vi "Tool_Playground.vi"() -> ()   [LabVIEW 2019]
uses:
  Parse/ParseVectorFile/Typedefs/PublicEvents--ParseVectorFile.ParsedData.ctl
  Parse/Image/SVGImage.lvclass
  Parse/ParsePaths/Path.lvclass
  Parse/Rectangle/Rectangle.lvclass
  Parse/Dot/Dot.lvclass
  Parse/ParseVectorFile/ParseVectorFile.lvclass
  C:/Program Files (x86)/National Instruments/LabVIEW 2019/vi.lib/JKI/JKI SMO/SMO/SMO.lvclass
  Settings/Rectangle Settings/Rectangle Settings.lvclass
  C:/Users/Albro/Documents/GitHub/AFM-Lithography/lvsrc/Classes/Settings/ObjectSettings/ObjectSettings.lvclass
  subVIs/typedefs/Schedule Types/Schedule--Constant.ctl
  Settings/ObjectSettings/ObjectSettings.lvclass/ObjectSettings.ctl
  Settings/Rectangle Settings/Rectangle Settings.lvclass/Rectangle Settings.ctl
  Settings/ObjectSettings/Accessors/Write Direction.vi
  Settings/ObjectSettings/Accessors/Write Enabled.vi
  Settings/ObjectSettings/Accessors/Write Resistance.vi
  Settings/ObjectSettings/Accessors/Write Speed Schedule.vi
  Settings/ObjectSettings/Accessors/Write Speed Settings.vi
  Settings/ObjectSettings/Accessors/Write Voltage Schedule.vi
  Settings/ObjectSettings/Accessors/Write Voltage Settings.vi
  Settings/Rectangle Settings/Accessors/Write Fill Orientation.vi
  Settings/Rectangle Settings/Accessors/Write Fill Spacing.vi
  Parse/Rectangle/Read Height.vi
  Settings/Rectangle Settings/Accessors/Read Fill Spacing.vi
  <vilib>/JKI/JKI SMO/SMO/SMO.lvclass
panel:
  out "ParsedData":T1
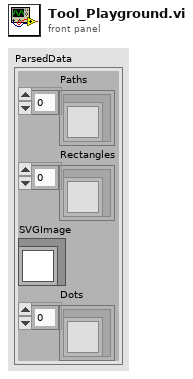
[diagram p1: front panel]
types:
  T1 = typedef "ParseVectorFile.lvclass/PublicEvents--ParseVectorFile.ParsedData.ctl" = cluster{"Paths":refnum<class "Path.lvclass">[], "Rectangles":refnum<class "Rectangle.lvclass">[], "SVGImage":refnum<class "SVGImage.lvclass">, "Dots":refnum<class "Dot.lvclass">[]}
  T2 = typedef "Schedule--Constant.ctl" = cluster{"Value":dbl}
  T3 = enum16{"Open", "Discharge Tip", "0 ohm", "100 kohm", "10 Mohm", "1 Gohm"}
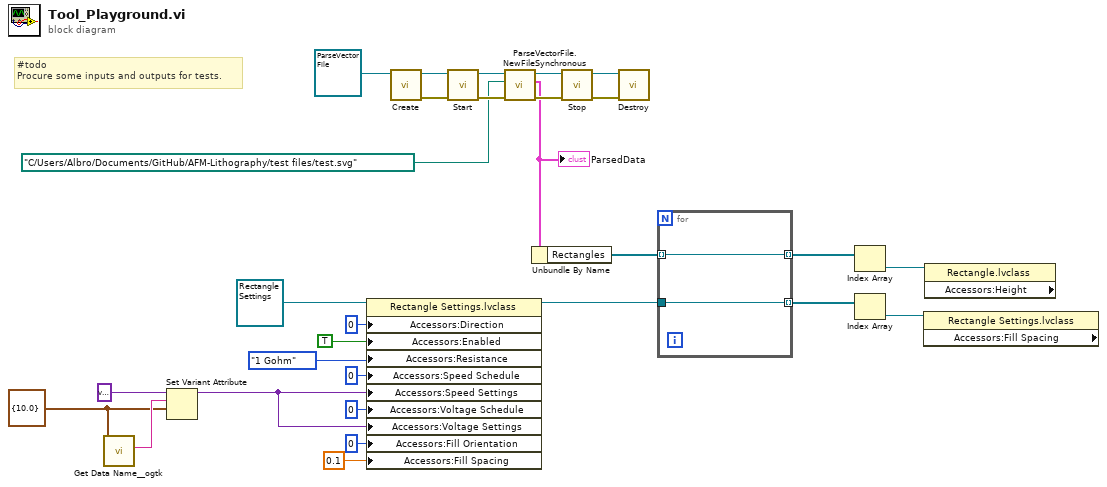
[diagram p0: block diagram]
diagram:
  w11 = T2 {"Value"=10.0} ("Constant")
  # "#todo\nProcure some inputs and outputs for tests."
  n1 = call <userlib>:"Get Data Name__ogtk.vi"("Data"=w11) -> ("Data Name"=w12:string)  [unwired: 8 in, 2 out]
  n2 = Set Variant Attribute(Variant=variant, name=w12, value=w11) -> (Variant out=w10:variant)  [unwired: 1 in, 2 out]
  n3 = property class="Rectangle Settings.lvclass"(reference=refnum<class "Rectangle Settings.lvclass"> refnum ("Rectangle Settings.lvclass"), "Accessors:Direction"=u16 0 ("Direction"), "Accessors:Enabled"=TRUE ("Enabled"), "Accessors:Resistance"=T3."1 Gohm" ("Resistance"), "Accessors:Speed Schedule"=u16 0 ("Speed Schedule"), "Accessors:Speed Settings"=w10, "Accessors:Voltage Schedule"=u16 0 ("Voltage Schedule"), "Accessors:Voltage Settings"=w10, "Accessors:Fill Orientation"=u16 0 ("Fill Orientation"), "Accessors:Fill Spacing"=0.1 ("Fill Spacing")) -> (reference out=w6:refnum<class "Rectangle Settings.lvclass">)  [unwired: 1 in, 1 out]
  n4 = call <vilib>:"Create.vi"("SMO"=refnum<class "ParseVectorFile.lvclass"> refnum ("ParseVectorFile out")) -> ("error out"=w28:errorcluster, "SMO out"=w29:refnum<class "ParseVectorFile.lvclass">)  [unwired: 8 in, 1 out]
  n5 = call <vilib>:"Start.vi"("error in (no error)"=w28, "SMO"=w29) -> ("error out"=w27:errorcluster, "SMO out"=w22:refnum<class "ParseVectorFile.lvclass">)  [unwired: 8 in]
  n6 = call "ParseVectorFile.NewFileSynchronous.vi"("error in (no error)"=w27, "Path"=path "C:/Users/Albro/Documents/GitHub/AFM-Lithography/test files/test.svg", "ParseVectorFile"=w22) -> ("error out"=w25:errorcluster, "ParsedData"=w9:T1, "ParseVectorFile out"=w26:refnum<class "ParseVectorFile.lvclass">)  [unwired: 6 in]
  "ParsedData" <- w9
  n7 = Unbundle By Name(w9) -> ("Rectangles"=w5:refnum<class "Rectangle.lvclass">[])
  n8 = call <vilib>:"Stop.vi"("error in (no error)"=w25, "SMO"=w26) -> ("error out"=w23:errorcluster, "SMO out"=w24:refnum<class "ParseVectorFile.lvclass">)  [unwired: 8 in]
  n9 = call <vilib>:"Destroy.vi"("error in (no error)"=w23, "SMO"=w24) -> ()  [unwired: 9 in, 1 out]
  n10 = for {
    tunnel: w6 -> [w31]
    tunnel: w5 -> [w30] mode=indexing
    tunnel: [w31] -> w3 mode=indexing
    tunnel: [w30] -> w4 mode=indexing
  }
  n11 = Index Array(array=w4) -> (element=w2:refnum<class "Rectangle.lvclass">)  [unwired: 1 in]
  n12 = Index Array(array=w3) -> (element=w1:refnum<class "Rectangle Settings.lvclass">)  [unwired: 1 in]
  n13 = property class="Rectangle Settings.lvclass" props=["Accessors:Fill Spacing"](reference=w1) -> ()  [unwired: 1 in, 3 out]
  n14 = property class="Rectangle.lvclass" props=["Accessors:Height"](reference=w2) -> ()  [unwired: 1 in, 3 out]
